vi "z[Lambda_tau,T,W,t_0]_Analytical.vi"(6 "t0":ext, 7 "Harmonic f":ext, 9 "W":ext, 10 "T":ext, 11 "tau":ext) -> (3 "z":cxt)   [LabVIEW 2019]
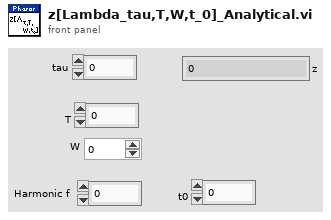
[diagram p1: front panel]
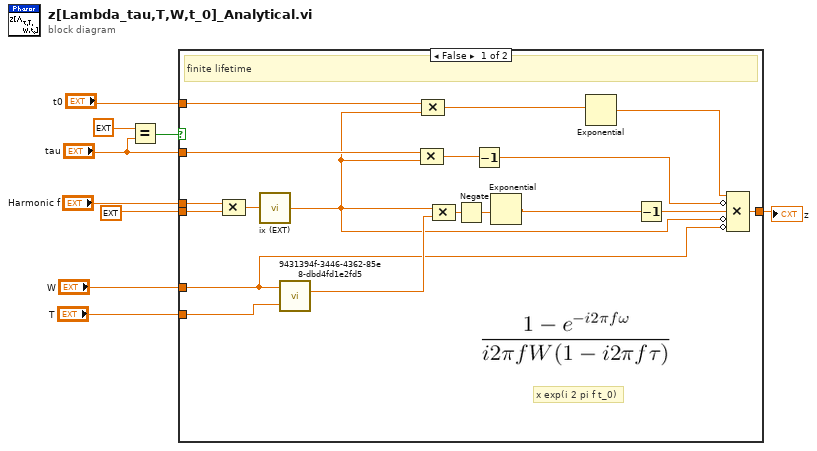
[diagram p0: block diagram]
diagram:
  n1 = Equal?(x=ext inf ("y"), y="tau") -> (x = y?=w2:bool)
  n2 = case shown="False" w2 {
    tunnel: "Harmonic f" -> [w27 _]
    tunnel: "T" -> [w26 _]
    tunnel: ext 6.283185307179586477 -> [w25 _]
    tunnel: "W" -> [w20 _]
    tunnel: [w16 _] -> w6
    tunnel: "t0" -> [w15 _]
    tunnel: "tau" -> [w12 _]
    frame False {
      # "x exp(i 2 pi f t_0)"
      # "finite lifetime"
      n3 = Compound Arithmetic op=MULTIPLY(w27, w25) -> (w11:ext)
      n4 = call "ix (EXT).vi"("x (1)"=w11) -> ("i.(x)"=w10:cxt)
      n5 = call "9431394f-3446-4362-85e8-dbd4fd1e2fd5.vi"("y"=w26, "x"=w20) -> ("x - E(x/y)y"=w23:ext)  [unwired: 1 out]
      n6 = Compound Arithmetic op=MULTIPLY(w12, w10) -> (w18:cxt)
      n7 = Compound Arithmetic op=MULTIPLY(w15, w10) -> (w14:cxt)
      n8 = Compound Arithmetic op=MULTIPLY(w10, w23) -> (w24:cxt)
      n9 = Negate(x=w24) -> (-x=w22:cxt)
      n10 = Decrement(x=w18) -> (x-1=w17:cxt)
      n11 = Exponential(1:w22) -> (0:w21:cxt)
      n12 = Exponential(1:w14) -> (0:w13:cxt)
      n13 = Decrement(x=w21) -> (x-1=w19:cxt)
      n14 = Compound Arithmetic op=MULTIPLY(w13, invert w17, w19, invert w10, invert w20) -> (w16:cxt)
    }
    frame True {
      # "infinite lifetime"
    }
  }
  "z" <- w6
